vi "Assign Pixel to Wing Sector (FPGA).vi"(0 "End Angle":u16, 2 "Right Wing?":bool, 3 "NumWingSectors":u8, 4 "Outter Radius":u16, 5 "Inner Radius":u16, 6 "Start Angle":u16, 7 "Hinge Y":u16, 8 "Hinge X":u16, 9 "Pixel Y":u16, 10 "Pixel X":u16) -> (1 "sector #":u8)   [LabVIEW 2013, in "FPGA Image Processing.lvlib"]
uses:
  FPGA Image Processing.lvlib
  <vilib>/rvi/FXPMathLib/FxpRectToPolar/subVIs/nifxpmath_RectToPolar_SimConfig.ctl
  <vilib>/rvi/FXPMathLib/FxpDiv/subVIs/nifxpmath_Div_SimConfig.ctl
  <vilib>/rvi/FXPMathLib/FxpRectToPolar/simVIs/DllFxpRectToPolarTemp_sub.vi
  <vilib>/rvi/FXPMathLib/FxpDiv/simVIs/DllFxpDivTemp_sub.vi
  <vilib>/rvi/FXPMathLib/FxpSub/XNode/nifxpmath_Sub.xnode
  <vilib>/rvi/FXPMathLib/FxpRectToPolar/XNode/nifxpmath_RectToPolar.xnode
  <vilib>/rvi/FXPMathLib/FxpDiv/XNode/nifxpmath_Div.xnode
  <vilib>/rvi/FXPMathLib/FxpAdd/XNode/nifxpmath_Add.xnode
  <vilib>/rvi/FXPMathLib/FxpMul/XNode/nifxpmath_Multiplier.xnode
  <vilib>/rvi/FXPMathLib/sim/FxpSim.dll
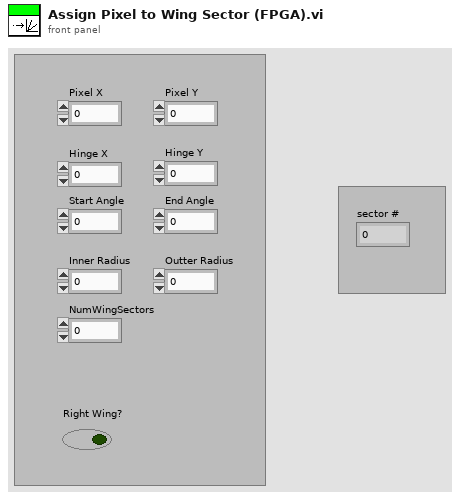
[diagram p1: front panel]
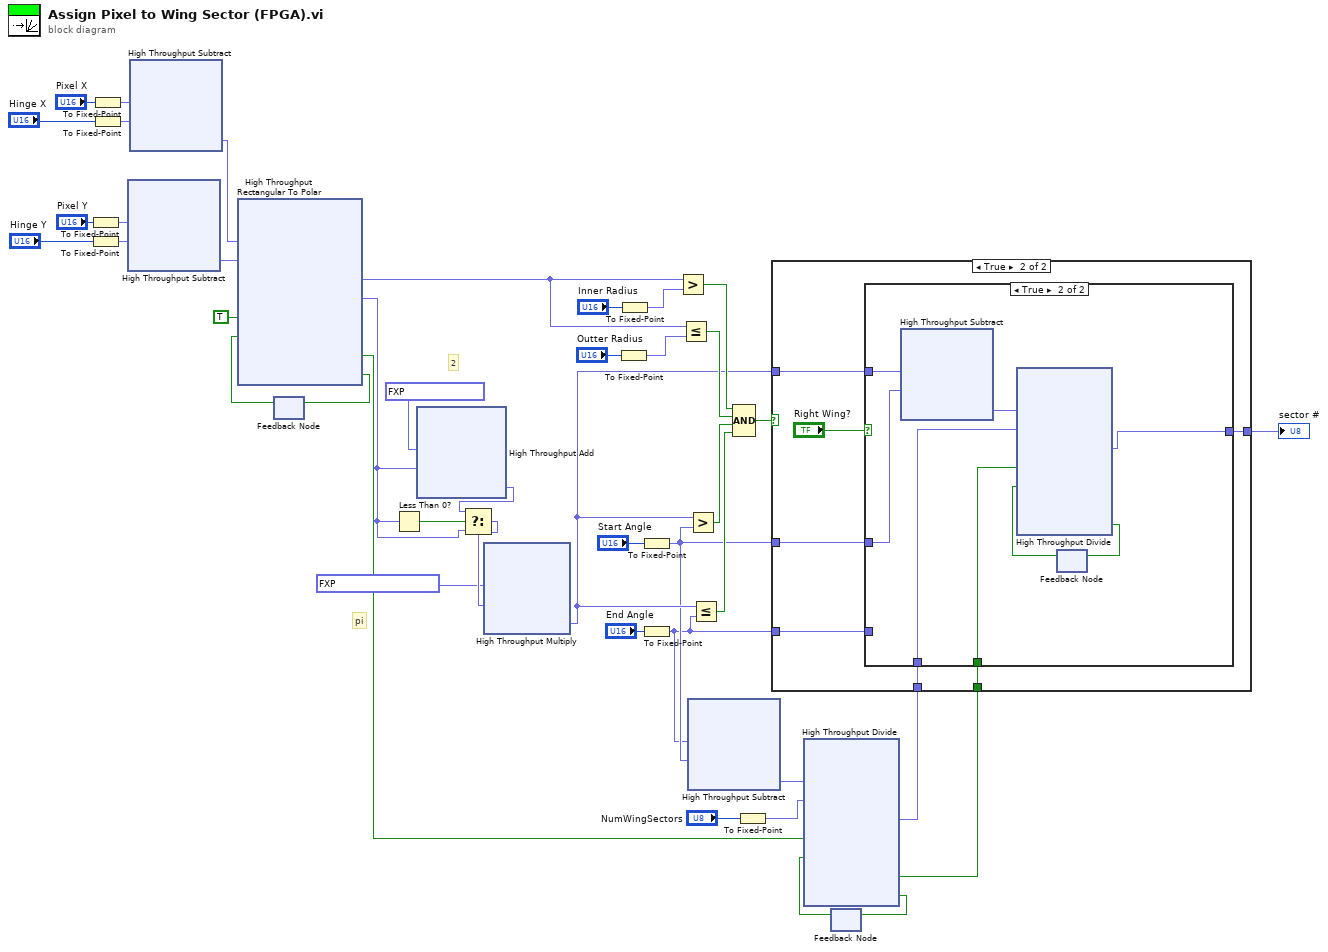
[diagram p0: block diagram]
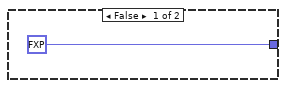
[diagram p2: hidden frame]
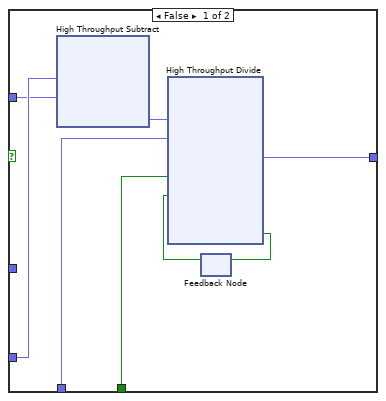
[diagram p3: hidden frame]
diagram:
  # "2"
  # "pi"
  n1 = To Fixed-Point(number="Pixel Y") -> (fixed-point=w38:fxp<+,16,16>)  [unwired: 1 in]
  n2 = To Fixed-Point(number="Hinge Y") -> (fixed-point=w37:fxp<+,16,16>)  [unwired: 1 in]
  n3 = To Fixed-Point(number="Pixel X") -> (fixed-point=w43:fxp<+,16,16>)  [unwired: 1 in]
  n4 = To Fixed-Point(number="Hinge X") -> (fixed-point=w41:fxp<+,16,16>)  [unwired: 1 in]
  n5 = xnode "High Throughput Subtract"("x"=w38, "y"=w37) -> ("x-y"=w34:fxp<+/-,18,18>)
  n6 = xnode "High Throughput Subtract"("x"=w43, "y"=w41) -> ("x-y"=w39:fxp<+/-,18,18>)
  n7 = feedback #1() -> (w5:bool)  [unwired: 1 in]
  n8 = xnode "High Throughput Rectangular To Polar"("x"=w39, "y"=w34, "input valid"=TRUE, "ready for output (T)"=w5) -> ("magnitude"=w31:fxp<+,18,18>, "phase (pi)"=w21:fxp<+/-,16,2>, "output valid"=w4:bool, "ready for input"=w6:bool)
  n9 = feedback-in #1(w6) -> ()
  n10 = Less Than 0?(x=w21) -> (x < 0?=w22:bool)
  n11 = xnode "High Throughput Add"("x"=fxp<+/-,16,2> 1.99993896484375 ("y"), "y"=w21) -> ("x+y"=w20:fxp<+/-,17,3>)
  n12 = Select(t=w20, s=w22, f=w21) -> (s? t:f=w18:fxp<+/-,17,3>)
  n13 = xnode "High Throughput Multiply"("x"=fxp<+,64,2> dbl? -8.87960937049345e+43, "y"=w18) -> ("x*y"=w16:fxp<+/-,64,5>)
  n14 = To Fixed-Point(number="Outter Radius") -> (fixed-point=w29:fxp<+,16,16>)  [unwired: 1 in]
  n15 = To Fixed-Point(number="Inner Radius") -> (fixed-point=w32:fxp<+,16,16>)  [unwired: 1 in]
  n16 = To Fixed-Point(number="Start Angle") -> (fixed-point=w15:fxp<+,16,16>)  [unwired: 1 in]
  n17 = To Fixed-Point(number="End Angle") -> (fixed-point=w9:fxp<+,16,16>)  [unwired: 1 in]
  n18 = Greater?(x=w31, y=w32) -> (0:w28:bool)
  n19 = Less Or Equal?(x=w31, y=w29) -> (x <= y?=w27:bool)
  n20 = Greater?(x=w16, y=w15) -> (0:w24:bool)
  n21 = xnode "High Throughput Subtract"("x"=w9, "y"=w15) -> ("x-y"=w14:fxp<+/-,18,18>)
  n22 = Less Or Equal?(x=w16, y=w9) -> (x <= y?=w23:bool)
  n23 = Compound Arithmetic op=AND(w28, w27, w24, w23) -> (w26:bool)
  n24 = To Fixed-Point(number="NumWingSectors") -> (fixed-point=w12:fxp<+,8,8>)  [unwired: 1 in]
  n25 = feedback #2() -> (w2:bool)  [unwired: 1 in]
  n26 = xnode "High Throughput Divide"("x"=w14, "y"=w12, "input valid"=w4, "ready for output (T)"=w2) -> ("x/y"=w11:fxp<+/-,18,18>, "output valid"=w1:bool, "ready for input"=w3:bool)
  n27 = case shown="True" w26 {
    tunnel: w16 -> [_ w50]
    tunnel: w15 -> [_ w49]
    tunnel: w11 -> [_ w48]
    tunnel: [fxp<+/-,64,18> 0.0 ("x/y") w47] -> w10
    tunnel: w9 -> [_ w46]
    tunnel: w1 -> [_ w45]
    frame False {
    }
    frame True {
      n28 = case shown="True" "Right Wing?" {
        tunnel: w50 -> [w58 w96]
        tunnel: w49 -> [_ w95]
        tunnel: w48 -> [w56 w93]
        tunnel: [w55 w92] -> w47
        tunnel: w46 -> [w59 _]
        tunnel: w45 -> [w52 w89]
        frame False {
          n29 = xnode "High Throughput Subtract"("x"=w59, "y"=w58) -> ("x-y"=w57:fxp<+/-,64,18>)
          n30 = feedback #3() -> (w53:bool)  [unwired: 1 in]
          n31 = xnode "High Throughput Divide"("x"=w57, "y"=w56, "input valid"=w52, "ready for output (T)"=w53) -> ("x/y"=w55:fxp<+/-,64,18>, "ready for input"=w54:bool)  [unwired: 1 out]
          n32 = feedback-in #3(w54) -> ()
        }
        frame True {
          n33 = xnode "High Throughput Subtract"("x"=w96, "y"=w95) -> ("x-y"=w94:fxp<+/-,64,18>)
          n34 = feedback #4() -> (w90:bool)  [unwired: 1 in]
          n35 = xnode "High Throughput Divide"("x"=w94, "y"=w93, "input valid"=w89, "ready for output (T)"=w90) -> ("x/y"=w92:fxp<+/-,64,18>, "ready for input"=w91:bool)  [unwired: 1 out]
          n36 = feedback-in #4(w91) -> ()
        }
      }
    }
  }
  "sector #" <- w10
  n37 = feedback-in #2(w3) -> ()
